vi "TAs StartTest (SubVI).vi"(8 "error in":errorcluster, 9 "Numeric":dbl format="%#_13g", 10 "Enum":enum16{"TA3", "TA2", "TA1"}(ring)) -> (0 "error out":errorcluster, 1 "String Out":string, 2 "Result":bool)   [LabVIEW 2017]
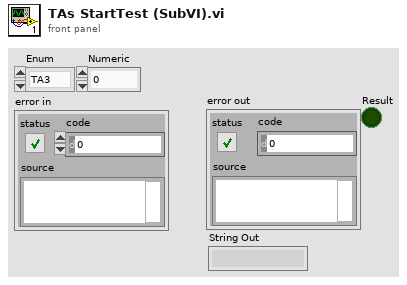
[diagram p1: front panel]
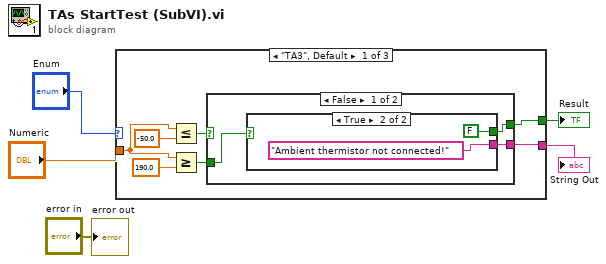
[diagram p0: block diagram]
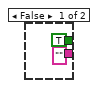
[diagram p2: hidden frame]
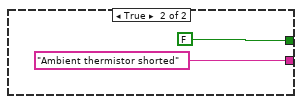
[diagram p3: hidden frame]
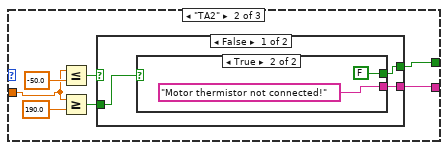
[diagram p4: hidden frame]
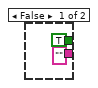
[diagram p5: hidden frame]
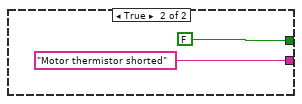
[diagram p6: hidden frame]
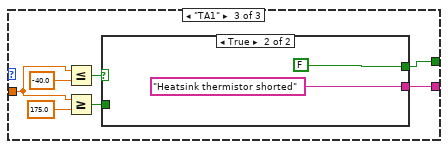
[diagram p7: hidden frame]
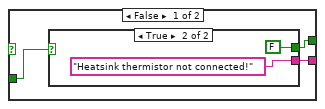
[diagram p8: hidden frame]
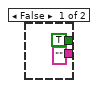
[diagram p9: hidden frame]
diagram:
  n1 = case shown="\"TA3\", Default" "Enum" {
    tunnel: [w8 w24 w40] -> w2
    tunnel: [w7 w23 w39] -> w1
    tunnel: "Numeric" -> [w6 w22 w38]
    frame "TA3", Default {
      n2 = Less Or Equal?(x=w6, y=-50.0) -> (x <= y?=w10:bool)
      n3 = Greater Or Equal?(x=w6, y=190.0) -> (x >= y?=w9:bool)
      n4 = case shown="False" w10 {
        tunnel: w9 -> [w15 _]
        tunnel: [w14 "Ambient thermistor shorted"] -> w7
        tunnel: [w13 FALSE] -> w8
        frame False {
          n5 = case shown="True" w15 {
            tunnel: ["" "Ambient thermistor not connected!"] -> w14
            tunnel: [TRUE FALSE] -> w13
            frame False {
            }
            frame True {
            }
          }
        }
        frame True {
        }
      }
    }
    frame "TA2" {
      n6 = Less Or Equal?(x=w22, y=-50.0) -> (x <= y?=w26:bool)
      n7 = Greater Or Equal?(x=w22, y=190.0) -> (x >= y?=w25:bool)
      n8 = case shown="False" w26 {
        tunnel: w25 -> [w31 _]
        tunnel: [w30 "Motor thermistor shorted"] -> w23
        tunnel: [w29 FALSE] -> w24
        frame False {
          n9 = case shown="True" w31 {
            tunnel: ["" "Motor thermistor not connected!"] -> w30
            tunnel: [TRUE FALSE] -> w29
            frame False {
            }
            frame True {
            }
          }
        }
        frame True {
        }
      }
    }
    frame "TA1" {
      n10 = Less Or Equal?(x=w38, y=-40.0) -> (x <= y?=w42:bool)
      n11 = Greater Or Equal?(x=w38, y=175.0) -> (x >= y?=w41:bool)
      n12 = case shown="True" w42 {
        tunnel: w41 -> [w47 _]
        tunnel: [w46 "Heatsink thermistor shorted"] -> w39
        tunnel: [w45 FALSE] -> w40
        frame False {
          n13 = case shown="True" w47 {
            tunnel: ["" "Heatsink thermistor not connected!"] -> w46
            tunnel: [TRUE FALSE] -> w45
            frame False {
            }
            frame True {
            }
          }
        }
        frame True {
        }
      }
    }
  }
  "Result" <- w2
  "String Out" <- w1
  "error out" <- "error in"
